vi "V4.vi"() -> ()   [LabVIEW 2020]
uses:
  <vilib>/Utility/NIReport.llb/Report Type.ctl
  <vilib>/Instr/_visa.llb/VISA Configure Serial Port (Instr).vi
  <vilib>/addons/_office/word.llb/Word Find & Replace (str).vi
  <vilib>/Utility/NIReport.llb/NI_report.lvclass
  <vilib>/Utility/NIReport.llb/NI_ReportGenerationCore.lvlib
  <vilib>/addons/_office/NI_ReportGenerationToolkit.lvlib
  <vilib>/Utility/NIReport.llb/Word/NI_Word.lvclass
panel:
  in  "?":bool
  in  "Buzzer":bool
  in  "Photoresistance":bool
  in  "Communication":bool
  in  "Infrarouge":bool
  in  "Ampoule":bool
  in  "Moteurs":bool
  in  "Initialisation":bool
  out "Booléen":bool=TRUE
  in  "Commande onglets":T1(tab)
  out "Derniere lettre":string
  out "Chaîne 2":string
  in  "COM":refnum<visa-resource-name>
  in  "Saisie :":i32
  out "Instructions :":string
  out "Vmax Chenilles":i32
  in  "Acquitemement":bool
  in  "Rotation sens direct":bool
  in  "Rotation sens indirecte":bool
  out "Rota Direct":bool=TRUE
  out "Rota Indirect":bool=TRUE
  in  "Allumé ?":bool
  out "INSTRUCTIONS":string
  in  "Bouton OK 2":bool
  out "Jauge":dbl(knob) scale=0.0..5.0
  in  "?":bool
  out "Instructions":string
  out "60 avant":dbl
  out "30 avant":dbl
  out "10 avant":dbl
  out "60 arriere":dbl
  out "30 arriere":dbl
  out "10 arriere":dbl
  out "Luminosité":dbl(slide) scale=0.0..100.0
  in  "?":bool
  out "INSTRUCTIONS":string
  out "Sombre":dbl
  out "Lumineux":dbl
  out "ambiant":dbl
  in  "Validation":bool
  in  "Etape suivante":bool
  out "avancer":bool
  out "reculer":bool
  out "Droite":bool
  out "gauche":bool
  out "bouton haut":bool
  out "bouton bas":bool
  out "Explication":string
  out "Graphe déroulant":dbl(graph)
  out "Db buzzer":dbl format="%#_13g"
  in  "Saisie Buzzer":dbl
  in  "Bouton OK Buzzer":bool
  out "INSTRUCTIONS":string
  in  "?":bool
  # "Brancher le capteur infrarouge sur l'entrée analogique  0. \nIl faudra l'avant en premier puis le deuxieme \n\nBrancher la photoresistance sur l'entrée analogique 3\n\nBrancher le récépteur de la télécomande sur l'entrée analogique 3. \nIl faurdra changer de canal afin de réaliser les différentes mesures \n\nPréparer également un tachymetre et un microphone."
  # "BIENVENUE SUR LE BANC DE TEST"
  # "Appuyer pour générer le rapport"
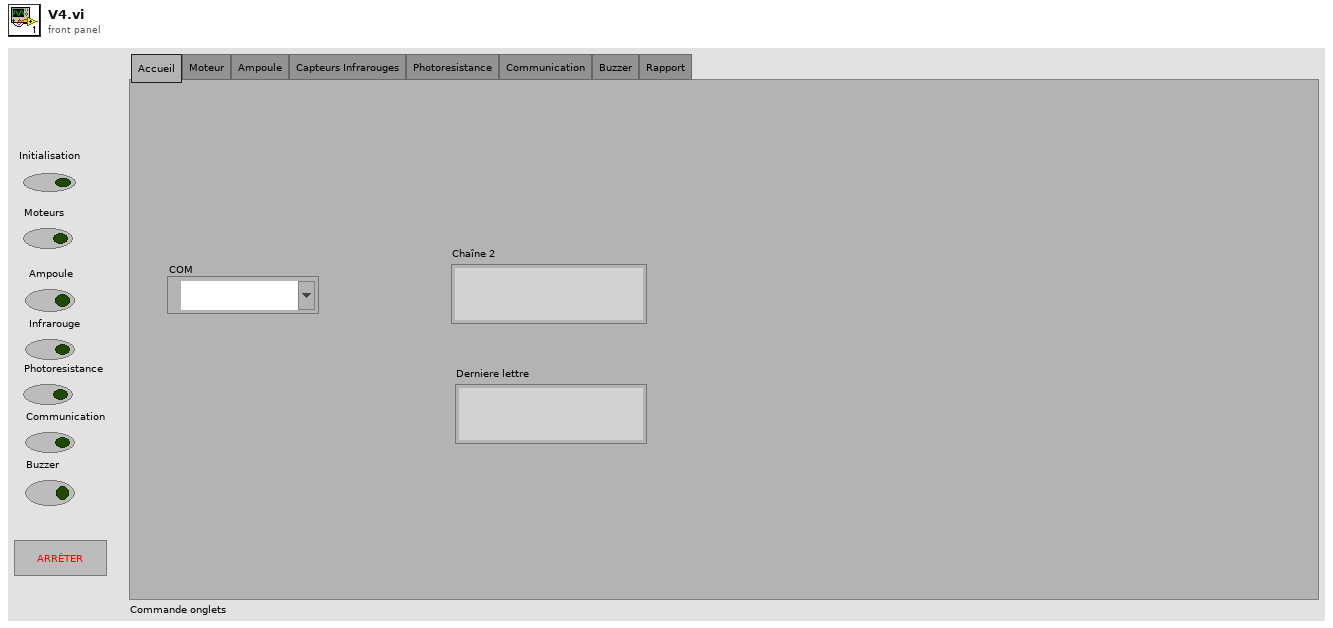
[diagram p1: front panel]
types:
  T1 = enum32{"Accueil", "Moteur", "Ampoule", "Capteurs Infrarouges", "Photoresistance", "Communication", "Buzzer", "Rapport"}
  T2 = typedef "NI_ReportGenerationCore.lvlib/Report Type.ctl" = enum16{"HTML", "Word", "Excel"}
  T3 = enum16{"maximized", "minimized", "normal", "no change"}
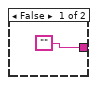
[diagram p3: hidden frame]
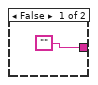
[diagram p4: hidden frame]
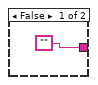
[diagram p5: hidden frame]
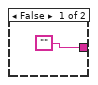
[diagram p6: hidden frame]
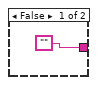
[diagram p7: hidden frame]
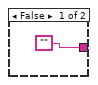
[diagram p8: hidden frame]
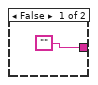
[diagram p9: hidden frame]
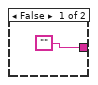
[diagram p10: hidden frame]
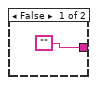
[diagram p11: hidden frame]
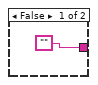
[diagram p12: hidden frame]
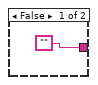
[diagram p13: hidden frame]
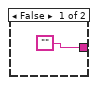
[diagram p14: hidden frame]
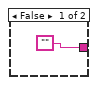
[diagram p15: hidden frame]
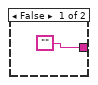
[diagram p16: hidden frame]
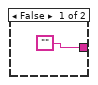
[diagram p17: hidden frame]
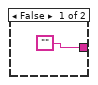
[diagram p18: hidden frame]
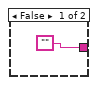
[diagram p19: hidden frame]
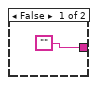
[diagram p20: hidden frame]
diagram:
  n1 = call-poly "VISA Configure Serial Port"("VISA resource name"="COM") -> ("VISA resource name out"=w3:refnum<visa-resource-name>, "error out"=w2:errorcluster)  [unwired: 13 in]
  n2 = while {
    shift-right: [w20] -> _
    shift-left: w3 -> [w17]
    shift-right: [w19] -> _
    shift-left: w2 -> [w18]
    tunnel: ["?"] -> w1
    stop <- w6 stop-if-true
    n3 = local read "Acquitemement"() -> (w10:bool)
    n4 = Or(x="?", y=w10) -> (x .or. y?=w9:bool)
    n5 = case shown="Faux" w9 {
      tunnel: ["" "X"] -> w8
      frame False {
      }
      frame True {
      }
    }
    n6 = case shown="Faux" "Infrarouge" {
      tunnel: ["" "D"] -> w34
      frame False {
      }
      frame True {
      }
    }
    n7 = case shown="Faux" "Photoresistance" {
      tunnel: ["" "E"] -> w33
      frame False {
      }
      frame True {
      }
    }
    n8 = case shown="Faux" "Communication" {
      tunnel: ["" "F"] -> w32
      frame False {
      }
      frame True {
      }
    }
    n9 = case shown="Faux" "Ampoule" {
      tunnel: ["" "C"] -> w35
      frame False {
      }
      frame True {
      }
    }
    n10 = case shown="Faux" "Moteurs" {
      tunnel: ["" "B"] -> w22
      frame False {
      }
      frame True {
      }
    }
    n11 = case shown="Faux" "Buzzer" {
      tunnel: ["" "G"] -> w31
      frame False {
      }
      frame True {
      }
    }
    n12 = case shown="Faux" "Initialisation" {
      tunnel: ["" "A"] -> w23
      frame False {
      }
      frame True {
      }
    }
    n13 = Concatenate Strings(w23, w22, w35, w34, w33, w32, w31, w8) -> (w12:string)
    n14 = case shown="\"F\"" w12 {
      frame "X", Default {
      }
      frame "A" {
        n15 = local write "Vmax Chenilles"(0) -> ()
        n16 = property on="Commande onglets" class="Onglet (strict)"("Value"=T1."Accueil" ("Commande onglets")) -> ()  [unwired: 2 in, 2 out]
      }
      frame "B" {
        n17 = property on="Commande onglets" class="Onglet (strict)"("Value"=T1."Moteur" ("Commande onglets")) -> ()  [unwired: 2 in, 2 out]
        n18 = case shown="Faux" TRUE {
          tunnel: [FALSE TRUE] -> w42
          tunnel: "entre valeur" -> [_ w51]
          tunnel: ["" w51] -> w40
          frame False {
          }
          frame True {
            n19 = Wait (ms)(milliseconds to wait=6000) -> ()  [unwired: 1 out]
            n20 = local write "Instructions :"("Attendre") -> ()
          }
        }
        n21 = local write "Instructions :"(w40) -> ()
        n22 = while {
          tunnel: ["Fini"] -> w43
          tunnel: w42 -> [_]
          stop <- "Acquitemement" stop-if-true
          n23 = local write "Rota Direct"("Rotation sens direct") -> ()
          n24 = local write "Rota Indirect"("Rotation sens indirecte") -> ()
          n25 = local write "Vmax Chenilles"("Saisie :") -> ()
        }
        "Instructions :" <- w43
      }
      frame "C" {
        n26 = property on="Commande onglets" class="Onglet (strict)"("Value"=T1."Ampoule" ("Commande onglets")) -> ()  [unwired: 2 in, 2 out]
        n27 = case shown="Vrai" TRUE {
          tunnel: [FALSE TRUE] -> w59
          tunnel: "Ampoule allumé ?" -> [_ w66]
          tunnel: ["" w66] -> w57
          frame False {
          }
          frame True {
            n28 = Wait (ms)(milliseconds to wait=4000) -> ()  [unwired: 1 out]
            n29 = local write "INSTRUCTIONS"("Attendre") -> ()
          }
        }
        n30 = local write "INSTRUCTIONS"(w57) -> ()
        n31 = while {
          tunnel: ["Fini"] -> w60
          tunnel: w59 -> [_]
          stop <- "Bouton OK 2" stop-if-true
          n32 = local write "Booléen"("Allumé ?") -> ()
        }
        "INSTRUCTIONS" <- w60
      }
      frame "D" {
        n33 = while {
          tunnel: [w123] -> w83
          tunnel: "Prise de valeur" -> [w123]
          tunnel: ["?"] -> w82
          stop <- "?" stop-if-true
          n34 = shared-variable "cRIO-9063\\Mod2\\AI0"() -> (→"Jauge":dbl)  [unwired: 1 in, 1 out]
          n35 = local write "Instructions"("Positionner le capteur avant a une distance de 60 cm") -> ()
        }
        n36 = local write "Instructions"(w83) -> ()
        n37 = case shown="Vrai" w82 {
          tunnel: [FALSE TRUE] -> w81
          frame False {
          }
          frame True {
            n38 = shared-variable "cRIO-9063\\Mod2\\AI0"() -> (w118:dbl)  [unwired: 1 in, 1 out]
            n39 = Wait (ms)(milliseconds to wait=150) -> ()  [unwired: 1 out]
            n40 = local write "60 avant"(w118) -> ()
          }
        }
        n41 = property on="Commande onglets" class="Onglet (strict)"("Value"=T1."Capteurs Infrarouges" ("Commande onglets")) -> ()  [unwired: 2 in, 2 out]
        n42 = while {
          tunnel: w81 -> [_]
          tunnel: [w126] -> w79
          stop <- w126 stop-if-true
          n43 = shared-variable "cRIO-9063\\Mod2\\AI0"() -> (w125:dbl)  [unwired: 1 in, 1 out]
          n44 = local read item#22() -> (w126:bool)
          n45 = local write "Jauge"(w125) -> ()
          n46 = local write "Instructions"("Positionner le capteur avant a une distance de 30 cm") -> ()
        }
        n47 = case shown="Vrai" w79 {
          tunnel: [FALSE TRUE] -> w78
          frame False {
          }
          frame True {
            n48 = shared-variable "cRIO-9063\\Mod2\\AI0"() -> (w114:dbl)  [unwired: 1 in, 1 out]
            n49 = Wait (ms)(milliseconds to wait=150) -> ()  [unwired: 1 out]
            n50 = local write "30 avant"(w114) -> ()
          }
        }
        n51 = while {
          tunnel: [w111] -> w80
          tunnel: w78 -> [_]
          stop <- w111 stop-if-true
          n52 = local read item#22() -> (w111:bool)
          n53 = shared-variable "cRIO-9063\\Mod2\\AI0"() -> (w110:dbl)  [unwired: 1 in, 1 out]
          n54 = local write "Jauge"(w110) -> ()
          n55 = local write "Instructions"("Positionner le capteur avant a une distance de 10 cm") -> ()
        }
        n56 = case shown="Vrai" w80 {
          tunnel: [FALSE TRUE] -> w76
          frame False {
          }
          frame True {
            n57 = shared-variable "cRIO-9063\\Mod2\\AI0"() -> (w107:dbl)  [unwired: 1 in, 1 out]
            n58 = Wait (ms)(milliseconds to wait=150) -> ()  [unwired: 1 out]
            n59 = local write "10 avant"(w107) -> ()
          }
        }
        n60 = while {
          tunnel: [w105] -> w77
          tunnel: w76 -> [_]
          stop <- w105 stop-if-true
          n61 = shared-variable "cRIO-9063\\Mod2\\AI1"() -> (w103:dbl)  [unwired: 1 in, 1 out]
          n62 = local read item#22() -> (w105:bool)
          n63 = local write "Jauge"(w103) -> ()
          n64 = local write "Instructions"("Positionner le capteur arriere a une distance de 60 cm") -> ()
        }
        n65 = case shown="Vrai" w77 {
          tunnel: [FALSE TRUE] -> w75
          frame False {
          }
          frame True {
            n66 = shared-variable "cRIO-9063\\Mod2\\AI1"() -> (w100:dbl)  [unwired: 1 in, 1 out]
            n67 = Wait (ms)(milliseconds to wait=150) -> ()  [unwired: 1 out]
            n68 = local write "60 arriere"(w100) -> ()
          }
        }
        n69 = while {
          tunnel: [w97] -> w74
          tunnel: w75 -> [_]
          stop <- w97 stop-if-true
          n70 = shared-variable "cRIO-9063\\Mod2\\AI1"() -> (w96:dbl)  [unwired: 1 in, 1 out]
          n71 = local read item#22() -> (w97:bool)
          n72 = local write "Jauge"(w96) -> ()
          n73 = local write "Instructions"("Positionner le capteur arriere a une distance de 30 cm") -> ()
        }
        n74 = case shown="Vrai" w74 {
          tunnel: [FALSE TRUE] -> w73
          frame False {
          }
          frame True {
            n75 = shared-variable "cRIO-9063\\Mod2\\AI1"() -> (w93:dbl)  [unwired: 1 in, 1 out]
            n76 = Wait (ms)(milliseconds to wait=150) -> ()  [unwired: 1 out]
            n77 = local write "30 arriere"(w93) -> ()
          }
        }
        n78 = while {
          tunnel: [w90] -> w72
          tunnel: w73 -> [_]
          stop <- w90 stop-if-true
          n79 = local read item#22() -> (w90:bool)
          n80 = shared-variable "cRIO-9063\\Mod2\\AI1"() -> (w89:dbl)  [unwired: 1 in, 1 out]
          n81 = local write "Jauge"(w89) -> ()
          n82 = local write "Instructions"("Positionner le capteur arriere a une distance de 10 cm") -> ()
        }
        n83 = case shown="Vrai" w72 {
          tunnel: ["" "Fini"] -> w70
          frame False {
          }
          frame True {
            n84 = shared-variable "cRIO-9063\\Mod2\\AI1"() -> (w86:dbl)  [unwired: 1 in, 1 out]
            n85 = Wait (ms)(milliseconds to wait=150) -> ()  [unwired: 1 out]
            n86 = local write "10 arriere"(w86) -> ()
          }
        }
        n87 = local write "Instructions"(w70) -> ()
      }
      frame "E" {
        n88 = property on="Commande onglets" class="Onglet (strict)"("Value"=T1."Photoresistance" ("Commande onglets")) -> ()  [unwired: 2 in, 2 out]
        n89 = while {
          tunnel: ["?"] -> w134
          stop <- "?" stop-if-true
          n90 = local write "INSTRUCTIONS"("Cacher la photoresistance et appuyer sur OK quand c'est bon") -> ()
        }
        n91 = case shown="Vrai" w134 {
          tunnel: [FALSE TRUE] -> w131
          frame False {
          }
          frame True {
            n92 = shared-variable "cRIO-9063\\Mod2\\AI3"() -> (w148:dbl)  [unwired: 1 in, 1 out]
            n93 = Wait (ms)(milliseconds to wait=150) -> ()  [unwired: 1 out]
            n94 = local write "Sombre"(w148) -> ()
          }
        }
        n95 = while {
          tunnel: [w145] -> w133
          tunnel: w131 -> [_]
          stop <- w145 stop-if-true
          n96 = local read item#32() -> (w145:bool)
          n97 = local write "INSTRUCTIONS"("éclairé la photorésistance") -> ()
        }
        n98 = case shown="Vrai" w133 {
          tunnel: [FALSE TRUE] -> w132
          frame False {
          }
          frame True {
            n99 = shared-variable "cRIO-9063\\Mod2\\AI3"() -> (w142:dbl)  [unwired: 1 in, 1 out]
            n100 = Wait (ms)(milliseconds to wait=150) -> ()  [unwired: 1 out]
            n101 = local write "Lumineux"(w142) -> ()
          }
        }
        n102 = while {
          stop <- FALSE stop-if-true
          n103 = shared-variable "cRIO-9063\\Mod2\\AI3"() -> (w153:dbl)  [unwired: 1 in, 1 out]
          n104 = Divide(x=w153, y=5) -> (x/y=w158:dbl)
          n105 = Multiply(x=w158, y=100) -> (x*y=→"Luminosité":dbl)
        }
        n106 = while {
          tunnel: [w139] -> w130
          tunnel: w132 -> [_]
          stop <- w139 stop-if-true
          n107 = local read item#32() -> (w139:bool)
          n108 = local write "INSTRUCTIONS"("éclairé a lumière ambiante") -> ()
        }
        n109 = case shown="Faux" w130 {
          tunnel: ["" "Fini"] -> w128
          frame False {
          }
          frame True {
            n110 = shared-variable "cRIO-9063\\Mod2\\AI3"() -> (w137:dbl)  [unwired: 1 in, 1 out]
            n111 = Wait (ms)(milliseconds to wait=150) -> ()  [unwired: 1 out]
            n112 = local write "ambiant"(w137) -> ()
          }
        }
        n113 = local write "INSTRUCTIONS"(w128) -> ()
      }
      frame "F" {
        n114 = while {
          tunnel: ["Etape suivante"] -> w171
          tunnel: TRUE -> [_]
          stop <- "Etape suivante" stop-if-true
          n115 = shared-variable "cRIO-9063\\Mod2\\AI2"() -> (w214:dbl)  [unwired: 1 in, 1 out]
          n116 = local write "Graphe déroulant"(w214) -> ()
          n117 = local write "Explication"(" Accelerer au max et appuyer sur OK") -> ()
        }
        n118 = property on="Commande onglets" class="Onglet (strict)"("Value"=T1."Communication" ("Commande onglets")) -> ()  [unwired: 2 in, 2 out]
        n119 = case shown="Vrai" w171 {
          tunnel: [FALSE TRUE] -> w170
          frame False {
          }
          frame True {
            n120 = local write "avancer"("Validation") -> ()
            n121 = Wait (ms)(milliseconds to wait=150) -> ()  [unwired: 1 out]
          }
        }
        n122 = while {
          tunnel: w170 -> [_]
          tunnel: [w212] -> w169
          stop <- w212 stop-if-true
          n123 = shared-variable "cRIO-9063\\Mod2\\AI2"() -> (w211:dbl)  [unwired: 1 in, 1 out]
          n124 = local read "Etape suivante"() -> (w212:bool)
          n125 = local write "Graphe déroulant"(w211) -> ()
          n126 = local write "Explication"(" decelerer  au max et appuyer sur OK") -> ()
        }
        n127 = case shown="Vrai" w169 {
          tunnel: [FALSE TRUE] -> w168
          frame False {
          }
          frame True {
            n128 = local read "Validation"() -> (w201:bool)
            n129 = local write "reculer"(w201) -> ()
            n130 = Wait (ms)(milliseconds to wait=150) -> ()  [unwired: 1 out]
          }
        }
        n131 = while {
          tunnel: w168 -> [_]
          tunnel: [w205] -> w167
          stop <- w205 stop-if-true
          n132 = local read "Etape suivante"() -> (w205:bool)
          n133 = shared-variable "cRIO-9063\\Mod2\\AI2"() -> (w204:dbl)  [unwired: 1 in, 1 out]
          n134 = local write "Graphe déroulant"(w204) -> ()
          n135 = local write "Explication"("aller à droite") -> ()
        }
        n136 = case shown="Vrai" w167 {
          tunnel: [FALSE TRUE] -> w166
          frame False {
          }
          frame True {
            n137 = local read "Validation"() -> (w197:bool)
            n138 = Wait (ms)(milliseconds to wait=150) -> ()  [unwired: 1 out]
            n139 = local write "Droite"(w197) -> ()
          }
        }
        n140 = while {
          tunnel: w166 -> [_]
          tunnel: [TRUE] -> _
          tunnel: [w193] -> w165
          stop <- w193 stop-if-true
          n141 = local read "Etape suivante"() -> (w193:bool)
          n142 = shared-variable "cRIO-9063\\Mod2\\AI2"() -> (w192:dbl)  [unwired: 1 in, 1 out]
          n143 = local write "Graphe déroulant"(w192) -> ()
          n144 = local write "Explication"("aller à gauche") -> ()
        }
        n145 = case shown="Vrai" w165 {
          tunnel: [FALSE TRUE] -> w164
          frame False {
          }
          frame True {
            n146 = local read "Validation"() -> (w189:bool)
            n147 = local write "gauche"(w189) -> ()
            n148 = Wait (ms)(milliseconds to wait=150) -> ()  [unwired: 1 out]
          }
        }
        n149 = while {
          tunnel: w164 -> [_]
          tunnel: [w186] -> w163
          stop <- w186 stop-if-true
          n150 = local read "Etape suivante"() -> (w186:bool)
          n151 = shared-variable "cRIO-9063\\Mod2\\AI2"() -> (w185:dbl)  [unwired: 1 in, 1 out]
          n152 = local write "Explication"("On va tester le bouton pour cela actionné le en haut et validé. ") -> ()
          n153 = local write "Graphe déroulant"(w185) -> ()
        }
        n154 = case shown="Vrai" w163 {
          tunnel: [FALSE TRUE] -> w162
          frame False {
          }
          frame True {
            n155 = local read "Validation"() -> (w182:bool)
            n156 = local write "bouton haut"(w182) -> ()
            n157 = Wait (ms)(milliseconds to wait=150) -> ()  [unwired: 1 out]
          }
        }
        n158 = while {
          tunnel: w162 -> [_]
          tunnel: [w179] -> w161
          stop <- w179 stop-if-true
          n159 = local read "Etape suivante"() -> (w179:bool)
          n160 = shared-variable "cRIO-9063\\Mod2\\AI2"() -> (w178:dbl)  [unwired: 1 in, 1 out]
          n161 = local write "Graphe déroulant"(w178) -> ()
          n162 = local write "Explication"("Actionner le bouton vers le bas et valider") -> ()
        }
        n163 = case shown="Vrai" w161 {
          tunnel: [FALSE TRUE] -> w160
          frame False {
          }
          frame True {
            n164 = local read "Validation"() -> (w175:bool)
            n165 = local write "bouton bas"(w175) -> ()
            n166 = Wait (ms)(milliseconds to wait=150) -> ()  [unwired: 1 out]
          }
        }
        n167 = case shown="Vrai" w160 {
          frame False {
          }
          frame True {
            n168 = local write "Explication"("Vous avez terminer") -> ()
          }
        }
      }
      frame "G" {
        n169 = property on="Commande onglets" class="Onglet (strict)"("Value"=T1."Buzzer" ("Commande onglets")) -> ()  [unwired: 2 in, 2 out]
        n170 = while {
          tunnel: TRUE -> [_]
          stop <- "Bouton OK Buzzer" stop-if-true
          n171 = local write "Db buzzer"("Saisie Buzzer") -> ()
          "INSTRUCTIONS" <- "Veulliez  intaller une application qui permet de mesurer le son. Puis entrer la valeur et appuyer sur OK"
        }
      }
      frame "H" {
      }
      frame "I" {
      }
    }
    n172 = String Length(string=w12) -> (length=w16:i32)
    n173 = Equal?(x=w16, y=1) -> (x = y?=w13:bool)
    n174 = case shown="Faux" w13 {
      tunnel: [w224 w225] -> w14
      tunnel: w12 -> [_ w225]
      frame False {
        n175 = local read "Chaîne 2"() -> (w224:string)
      }
      frame True {
        "Chaîne 2" <- w225
      }
    }
    "Derniere lettre" <- w14
    n176 = Wait Until Next ms Multiple(millisecond multiple=100) -> ()  [unwired: 1 out]
    n177 = VISA Write(VISA resource name=w17, write buffer=w12, error in (no error)=w18) -> (VISA resource name out=w20:refnum<visa-resource-name>, error out=w19:errorcluster)  [unwired: 1 out]
    n178 = Or(x="?", y=FALSE) -> (x .or. y?=w6:bool)
  }
  n179 = case shown="Vrai" w1 {
    frame False {
    }
    frame True {
      n180 = Get Date/Time String(date format (0)=enum16{"short", "long", "abbreviated"}."short" ("format de date (0)"), seconds (now)=timestamp(0 s since 1904-01-01) ("horodatage"), want seconds? (F)=FALSE ("secondes ? (F)")) -> (date string=w331:string, time string=w289:string)
      n181 = local read "30 avant"() -> (w411:dbl)
      n182 = call <vilib>:"Create Report.vi"("window state (normal)"=T3."normal", "report type"=Report_Type."Word", "template (empty)"=path "P:/Saé/RapportDeTestVide.docx") -> ("report out"=w333:refnum<class "NI_report.lvclass">)  [unwired: 11 in, 1 out]
      n183 = Number To Decimal String(number=w411) -> (decimal integer string=w287:string)  [unwired: 1 in]
      n184 = call-poly <vilib>:"Word Find & Replace.vi"("report in"=w333, "find what?"="DATE", "replace with"=w331) -> ("report out"=w330:refnum<class "NI_report.lvclass">)  [unwired: 10 in, 2 out]
      n185 = local read "10 avant"() -> (w410:dbl)
      n186 = local read "60 avant"() -> (w344:dbl)
      n187 = Number To Decimal String(number=w410) -> (decimal integer string=w286:string)  [unwired: 1 in]
      n188 = local read "Vmax Chenilles"() -> (w421:i32)
      n189 = call-poly <vilib>:"Word Find & Replace.vi"("report in"=w330, "find what?"="HEURE", "replace with"=w289) -> ("report out"=w329:refnum<class "NI_report.lvclass">)  [unwired: 10 in, 2 out]
      n190 = Less Or Equal?(x=w344, y=0.6) -> (x <= y?=w368:bool)
      n191 = Greater Or Equal?(x=w344, y=0.5) -> (x >= y?=w369:bool)
      n192 = local read "60 arriere"() -> (w409:dbl)
      n193 = local read "Rota Indirect"() -> (w419:bool)
      n194 = local read "Rota Direct"() -> (w420:bool)
      n195 = And(x=w369, y=w368) -> (x .and. y?=w367:bool)
      n196 = Number To Decimal String(number=w421) -> (decimal integer string=w291:string)  [unwired: 1 in]
      n197 = Number To Decimal String(number=w409) -> (decimal integer string=w283:string)  [unwired: 1 in]
      n198 = case shown="Vrai" w367 {
        tunnel: ["" "X"] -> w257
        frame False {
        }
        frame True {
        }
      }
      n199 = And(x=w420, y=w419) -> (x .and. y?=w418:bool)
      n200 = call-poly <vilib>:"Word Find & Replace.vi"("report in"=w329, "find what?"="Mvmes", "replace with"=w291) -> ("report out"=w328:refnum<class "NI_report.lvclass">)  [unwired: 10 in, 2 out]
      n201 = case shown="Vrai" w418 {
        tunnel: ["" "X"] -> w293
        frame False {
        }
        frame True {
        }
      }
      n202 = local read "30 arriere"() -> (w408:dbl)
      n203 = local read "30 avant"() -> (w343:dbl)
      n204 = local read "Vmax Chenilles"() -> (w391:i32)
      n205 = Number To Decimal String(number=w408) -> (decimal integer string=w281:string)  [unwired: 1 in]
      n206 = local read "Booléen"() -> (w417:bool)
      n207 = call-poly <vilib>:"Word Find & Replace.vi"("report in"=w328, "find what?"="Cms", "replace with"=w293) -> ("report out"=w327:refnum<class "NI_report.lvclass">)  [unwired: 10 in, 2 out]
      n208 = Less Or Equal?(x=w343, y=1.1) -> (x <= y?=w363:bool)
      n209 = Greater Or Equal?(x=w343, y=0.9) -> (x >= y?=w364:bool)
      n210 = local read "10 arriere"() -> (w407:dbl)
      n211 = And(x=w364, y=w363) -> (x .and. y?=w362:bool)
      n212 = case shown="Vrai" w417 {
        tunnel: ["" "X"] -> w295
        frame False {
        }
        frame True {
        }
      }
      n213 = Less Or Equal?(x=w391, y=200) -> (x <= y?=w398:bool)
      n214 = Greater Or Equal?(x=w391, y=100) -> (x >= y?=w399:bool)
      n215 = case shown="Vrai" w362 {
        tunnel: ["" "X"] -> w259
        frame False {
        }
        frame True {
        }
      }
      n216 = Number To Decimal String(number=w407) -> (decimal integer string=w279:string)  [unwired: 1 in]
      n217 = And(x=w399, y=w398) -> (x .and. y?=w395:bool)
      n218 = call-poly <vilib>:"Word Find & Replace.vi"("report in"=w327, "find what?"="Ca", "replace with"=w295) -> ("report out"=w326:refnum<class "NI_report.lvclass">)  [unwired: 10 in, 2 out]
      n219 = case shown="Vrai" w395 {
        tunnel: ["" "X"] -> w277
        frame False {
        }
        frame True {
        }
      }
      n220 = local read "10 avant"() -> (w342:dbl)
      n221 = local read "Db buzzer"() -> (w416:dbl)
      n222 = Number To Decimal String(number=w416) -> (decimal integer string=w297:string)  [unwired: 1 in]
      n223 = local read "Db buzzer"() -> (w390:dbl)
      n224 = Less Or Equal?(x=w342, y=2.75) -> (x <= y?=w358:bool)
      n225 = Greater Or Equal?(x=w342, y=2.25) -> (x >= y?=w359:bool)
      n226 = call-poly <vilib>:"Word Find & Replace.vi"("report in"=w326, "find what?"="Buz1", "replace with"=w297) -> ("report out"=w325:refnum<class "NI_report.lvclass">)  [unwired: 10 in, 2 out]
      n227 = And(x=w359, y=w358) -> (x .and. y?=w357:bool)
      n228 = local read "Sombre"() -> (w415:dbl)
      n229 = case shown="Vrai" w357 {
        tunnel: ["" "X"] -> w261
        frame False {
        }
        frame True {
        }
      }
      n230 = Less Or Equal?(x=w390, y=75.0) -> (x <= y?=w393:bool)
      n231 = Greater Or Equal?(x=w390, y=60.0) -> (x >= y?=w394:bool)
      n232 = Number To Decimal String(number=w415) -> (decimal integer string=w299:string)  [unwired: 1 in]
      n233 = And(x=w394, y=w393) -> (x .and. y?=w392:bool)
      n234 = local read "60 arriere"() -> (w336:dbl)
      n235 = case shown="Vrai" w392 {
        tunnel: ["" "X"] -> w275
        frame False {
        }
        frame True {
        }
      }
      n236 = call-poly <vilib>:"Word Find & Replace.vi"("report in"=w325, "find what?"="Phon", "replace with"=w299) -> ("report out"=w324:refnum<class "NI_report.lvclass">)  [unwired: 10 in, 2 out]
      n237 = local read "Lumineux"() -> (w414:dbl)
      n238 = Less Or Equal?(x=w336, y=0.6) -> (x <= y?=w353:bool)
      n239 = Greater Or Equal?(x=w336, y=0.5) -> (x >= y?=w354:bool)
      n240 = local read "Sombre"() -> (w372:dbl)
      n241 = Number To Decimal String(number=w414) -> (decimal integer string=w301:string)  [unwired: 1 in]
      n242 = And(x=w354, y=w353) -> (x .and. y?=w352:bool)
      n243 = call-poly <vilib>:"Word Find & Replace.vi"("report in"=w324, "find what?"="Phoj", "replace with"=w301) -> ("report out"=w323:refnum<class "NI_report.lvclass">)  [unwired: 10 in, 2 out]
      n244 = local read "ambiant"() -> (w413:dbl)
      n245 = case shown="Vrai" w352 {
        tunnel: ["" "X"] -> w263
        frame False {
        }
        frame True {
        }
      }
      n246 = Less Or Equal?(x=w372, y=0.3) -> (x <= y?=w386:bool)
      n247 = Greater Or Equal?(x=w372, y=0.0) -> (x >= y?=w387:bool)
      n248 = Number To Decimal String(number=w413) -> (decimal integer string=w303:string)  [unwired: 1 in]
      n249 = And(x=w387, y=w386) -> (x .and. y?=w385:bool)
      n250 = local read "30 arriere"() -> (w335:dbl)
      n251 = local read "avancer"() -> (w406:bool)
      n252 = case shown="Vrai" w385 {
        tunnel: ["" "X"] -> w273
        frame False {
        }
        frame True {
        }
      }
      n253 = call-poly <vilib>:"Word Find & Replace.vi"("report in"=w323, "find what?"="Phoa", "replace with"=w303) -> ("report out"=w322:refnum<class "NI_report.lvclass">)  [unwired: 10 in, 2 out]
      n254 = Less Or Equal?(x=w335, y=1.1) -> (x <= y?=w348:bool)
      n255 = Greater Or Equal?(x=w335, y=0.9) -> (x >= y?=w349:bool)
      n256 = case shown="Vrai" w406 {
        tunnel: ["" "X"] -> w305
        frame False {
        }
        frame True {
        }
      }
      n257 = local read "Lumineux"() -> (w371:dbl)
      n258 = And(x=w349, y=w348) -> (x .and. y?=w347:bool)
      n259 = call-poly <vilib>:"Word Find & Replace.vi"("report in"=w322, "find what?"="Ccj", "replace with"=w305) -> ("report out"=w321:refnum<class "NI_report.lvclass">)  [unwired: 10 in, 2 out]
      n260 = local read "reculer"() -> (w405:bool)
      n261 = case shown="Vrai" w347 {
        tunnel: ["" "X"] -> w265
        frame False {
        }
        frame True {
        }
      }
      n262 = Less Or Equal?(x=w371, y=5.2) -> (x <= y?=w381:bool)
      n263 = Greater Or Equal?(x=w371, y=4.8) -> (x >= y?=w382:bool)
      n264 = case shown="Vrai" w405 {
        tunnel: ["" "X"] -> w307
        frame False {
        }
        frame True {
        }
      }
      n265 = And(x=w382, y=w381) -> (x .and. y?=w380:bool)
      n266 = local read "Droite"() -> (w404:bool)
      n267 = local read "10 arriere"() -> (w334:dbl)
      n268 = case shown="Vrai" w380 {
        tunnel: ["" "X"] -> w271
        frame False {
        }
        frame True {
        }
      }
      n269 = call-poly <vilib>:"Word Find & Replace.vi"("report in"=w321, "find what?"="Ccr", "replace with"=w307) -> ("report out"=w320:refnum<class "NI_report.lvclass">)  [unwired: 10 in, 2 out]
      n270 = case shown="Vrai" w404 {
        tunnel: ["" "X"] -> w309
        frame False {
        }
        frame True {
        }
      }
      n271 = local read "ambiant"() -> (w370:dbl)
      n272 = Less Or Equal?(x=w334, y=2.75) -> (x <= y?=w340:bool)
      n273 = Greater Or Equal?(x=w334, y=2.25) -> (x >= y?=w341:bool)
      n274 = And(x=w341, y=w340) -> (x .and. y?=w339:bool)
      n275 = local read "gauche"() -> (w403:bool)
      n276 = call-poly <vilib>:"Word Find & Replace.vi"("report in"=w320, "find what?"="Ccd", "replace with"=w309) -> ("report out"=w319:refnum<class "NI_report.lvclass">)  [unwired: 10 in, 2 out]
      n277 = case shown="Vrai" w339 {
        tunnel: ["" "X"] -> w267
        frame False {
        }
        frame True {
        }
      }
      n278 = Less Or Equal?(x=w370, y=4.8) -> (x <= y?=w376:bool)
      n279 = Greater Or Equal?(x=w370, y=0.3) -> (x >= y?=w377:bool)
      n280 = local read "bouton haut"() -> (w402:bool)
      n281 = local read "bouton bas"() -> (w400:bool)
      n282 = case shown="Vrai" w403 {
        tunnel: ["" "X"] -> w311
        frame False {
        }
        frame True {
        }
      }
      n283 = And(x=w377, y=w376) -> (x .and. y?=w375:bool)
      n284 = case shown="Vrai" w375 {
        tunnel: ["" "X"] -> w269
        frame False {
        }
        frame True {
        }
      }
      n285 = And(x=w402, y=w400) -> (x .and. y?=w401:bool)
      n286 = call-poly <vilib>:"Word Find & Replace.vi"("report in"=w319, "find what?"="Ccg", "replace with"=w311) -> ("report out"=w318:refnum<class "NI_report.lvclass">)  [unwired: 10 in, 2 out]
      n287 = case shown="Vrai" w401 {
        tunnel: ["" "X"] -> w313
        frame False {
        }
        frame True {
        }
      }
      n288 = call-poly <vilib>:"Word Find & Replace.vi"("report in"=w318, "find what?"="Ccb", "replace with"=w313) -> ("report out"=w317:refnum<class "NI_report.lvclass">)  [unwired: 10 in, 2 out]
      n289 = local read "60 avant"() -> (w412:dbl)
      n290 = Number To Decimal String(number=w412) -> (decimal integer string=w315:string)  [unwired: 1 in]
      n291 = call-poly <vilib>:"Word Find & Replace.vi"("report in"=w317, "find what?"="Irav60", "replace with"=w315) -> ("report out"=w256:refnum<class "NI_report.lvclass">)  [unwired: 10 in, 2 out]
      n292 = call-poly <vilib>:"Word Find & Replace.vi"("report in"=w256, "find what?"="Irav30", "replace with"=w287) -> ("report out"=w255:refnum<class "NI_report.lvclass">)  [unwired: 10 in, 2 out]
      n293 = call-poly <vilib>:"Word Find & Replace.vi"("report in"=w255, "find what?"="Irav10", "replace with"=w286) -> ("report out"=w254:refnum<class "NI_report.lvclass">)  [unwired: 10 in, 2 out]
      n294 = call-poly <vilib>:"Word Find & Replace.vi"("report in"=w254, "find what?"="Irar60", "replace with"=w283) -> ("report out"=w253:refnum<class "NI_report.lvclass">)  [unwired: 10 in, 2 out]
      n295 = call-poly <vilib>:"Word Find & Replace.vi"("report in"=w253, "find what?"="Irar30", "replace with"=w281) -> ("report out"=w252:refnum<class "NI_report.lvclass">)  [unwired: 10 in, 2 out]
      n296 = call-poly <vilib>:"Word Find & Replace.vi"("report in"=w252, "find what?"="Irar10", "replace with"=w279) -> ("report out"=w251:refnum<class "NI_report.lvclass">)  [unwired: 10 in, 2 out]
      n297 = call-poly <vilib>:"Word Find & Replace.vi"("report in"=w251, "find what?"="Cmv", "replace with"=w277) -> ("report out"=w250:refnum<class "NI_report.lvclass">)  [unwired: 10 in, 2 out]
      n298 = call-poly <vilib>:"Word Find & Replace.vi"("report in"=w250, "find what?"="Cb", "replace with"=w275) -> ("report out"=w249:refnum<class "NI_report.lvclass">)  [unwired: 10 in, 2 out]
      n299 = call-poly <vilib>:"Word Find & Replace.vi"("report in"=w249, "find what?"="Cn", "replace with"=w273) -> ("report out"=w248:refnum<class "NI_report.lvclass">)  [unwired: 10 in, 2 out]
      n300 = call-poly <vilib>:"Word Find & Replace.vi"("report in"=w248, "find what?"="Cj", "replace with"=w271) -> ("report out"=w247:refnum<class "NI_report.lvclass">)  [unwired: 10 in, 2 out]
      n301 = call-poly <vilib>:"Word Find & Replace.vi"("report in"=w247, "find what?"="Cpa", "replace with"=w269) -> ("report out"=w246:refnum<class "NI_report.lvclass">)  [unwired: 10 in, 2 out]
      n302 = call-poly <vilib>:"Word Find & Replace.vi"("report in"=w246, "find what?"="Cia6", "replace with"=w257) -> ("report out"=w245:refnum<class "NI_report.lvclass">)  [unwired: 10 in, 2 out]
      n303 = call-poly <vilib>:"Word Find & Replace.vi"("report in"=w245, "find what?"="Cia3", "replace with"=w259) -> ("report out"=w244:refnum<class "NI_report.lvclass">)  [unwired: 10 in, 2 out]
      n304 = call-poly <vilib>:"Word Find & Replace.vi"("report in"=w244, "find what?"="Cia1", "replace with"=w261) -> ("report out"=w243:refnum<class "NI_report.lvclass">)  [unwired: 10 in, 2 out]
      n305 = call-poly <vilib>:"Word Find & Replace.vi"("report in"=w243, "find what?"="Cir6", "replace with"=w263) -> ("report out"=w242:refnum<class "NI_report.lvclass">)  [unwired: 10 in, 2 out]
      n306 = call-poly <vilib>:"Word Find & Replace.vi"("report in"=w242, "find what?"="Cir3", "replace with"=w265) -> ("report out"=w241:refnum<class "NI_report.lvclass">)  [unwired: 10 in, 2 out]
      n307 = call-poly <vilib>:"Word Find & Replace.vi"("report in"=w241, "find what?"="Cir1", "replace with"=w267) -> ("report out"=w240:refnum<class "NI_report.lvclass">)  [unwired: 10 in, 2 out]
      n308 = call-dynamic "Save Report to File.vi"("report in"=w240, "report file path"=path "P:/Saé/RapportDeTestRemplie.docx") -> ()  [unwired: 12 in, 2 out]
    }
  }
